vi "Invert Build Type.vi"(8 "error in (no error)":errorcluster, 11 "Build Type String":string) -> (0 "error out":errorcluster, 2 "Inverted Build Type":string, 3 "Build Type String out (dup)":string)   [LabVIEW 2019, in "NIPKG Naming.lvlib"]
doc: "Produces the opposite (Debug/Release) build type string."
uses:
  NIPKG Naming.lvlib
  <vilib>/ErrorRing/Error Ring.xnode
  <vilib>/Utility/error.llb/Error Cluster From Error Code.vi
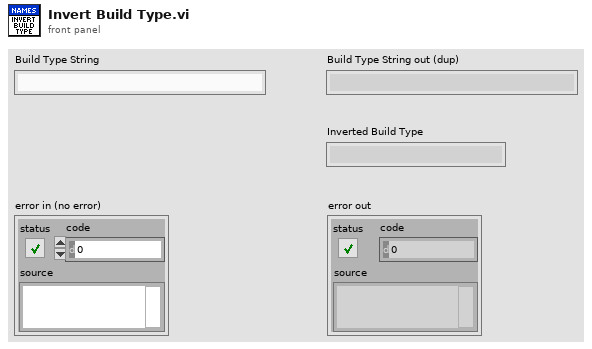
[diagram p1: front panel]
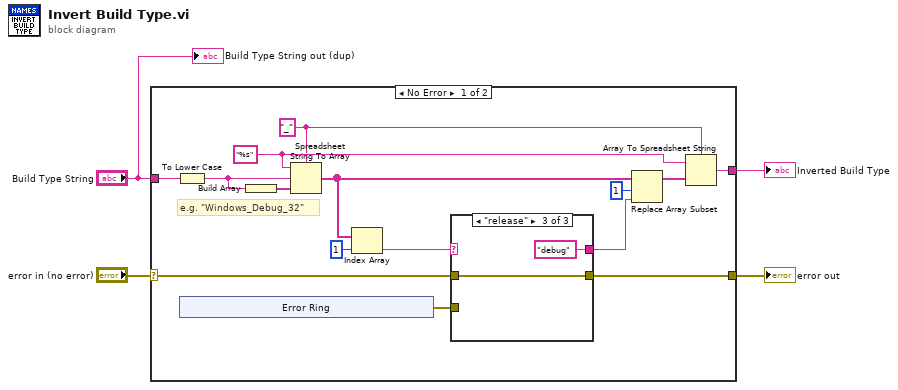
[diagram p0: block diagram]
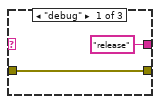
[diagram p2: hidden frame]
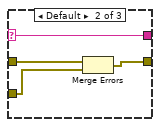
[diagram p3: hidden frame]
diagram:
  n1 = case shown="No Error" "error in (no error)" {
    selector: "error in (no error)" -> [w16 w32]
    tunnel: "Build Type String" -> [w17 _]
    tunnel: [w10 w32] -> w3
    tunnel: [w6 _] -> w1
    frame No Error {
      w7 = "_" ("delimiter (Tab)")
      w8 = "%s" ("format string")
      # "e.g. \"Windows_Debug_32\""
      n2 = To Lower Case(string=w17) -> (all lower case string=w18:string)
      n3 = xnode "Error Ring"() -> ("error out"=w5:errorcluster)
      n4 = Build Array(w18) -> (w19:string[])
      n5 = Spreadsheet String To Array(delimiter (Tab)=w7, format string=w8, spreadsheet string=w18, array type (2D Dbl)=w19) -> (array=w13:string[])
      n6 = Index Array(array=w13, index=1) -> (element=w14:string)
      n7 = case shown="\"release\"" w14 {
        selector: w14 -> [_ w29 _]
        tunnel: w16 -> [w24 w28 w30]
        tunnel: ["release" w29 "debug"] -> w11
        tunnel: [w24 w27 w30] -> w10
        tunnel: w5 -> [_ w26 _]
        frame "debug" {
        }
        frame Default {
          n8 = Merge Errors(w28, w26) -> (w27:errorcluster)
        }
        frame "release" {
        }
      }
      n9 = Replace Array Subset(array=w13, new element=w11, index=1) -> (w9:string[])
      n10 = Array To Spreadsheet String(delimiter (Tab)=w7, array=w9, 3:w8) -> (spreadsheet string=w6:string)
    }
    frame Error {
    }
  }
  "Inverted Build Type" <- w1
  "error out" <- w3
  "Build Type String out (dup)" <- "Build Type String"
